vi "j_GetJoystickSignal.vi"(5 "RelJoyPos In":T1, 6 "NewJoystButtInfo":T2, 7 "NewJoystAxisInfo":T4, 8 "OldJoystButtInfo":T2, 9 "OldJoystickOffset":T3) -> (0 "MoveZ":bool, 1 "MoveXY":bool, 2 "Joystick Offset":T3, 3 "RelJoyPos":T1, 4 "TalkToMotors?":bool)   [LabVIEW 2014]
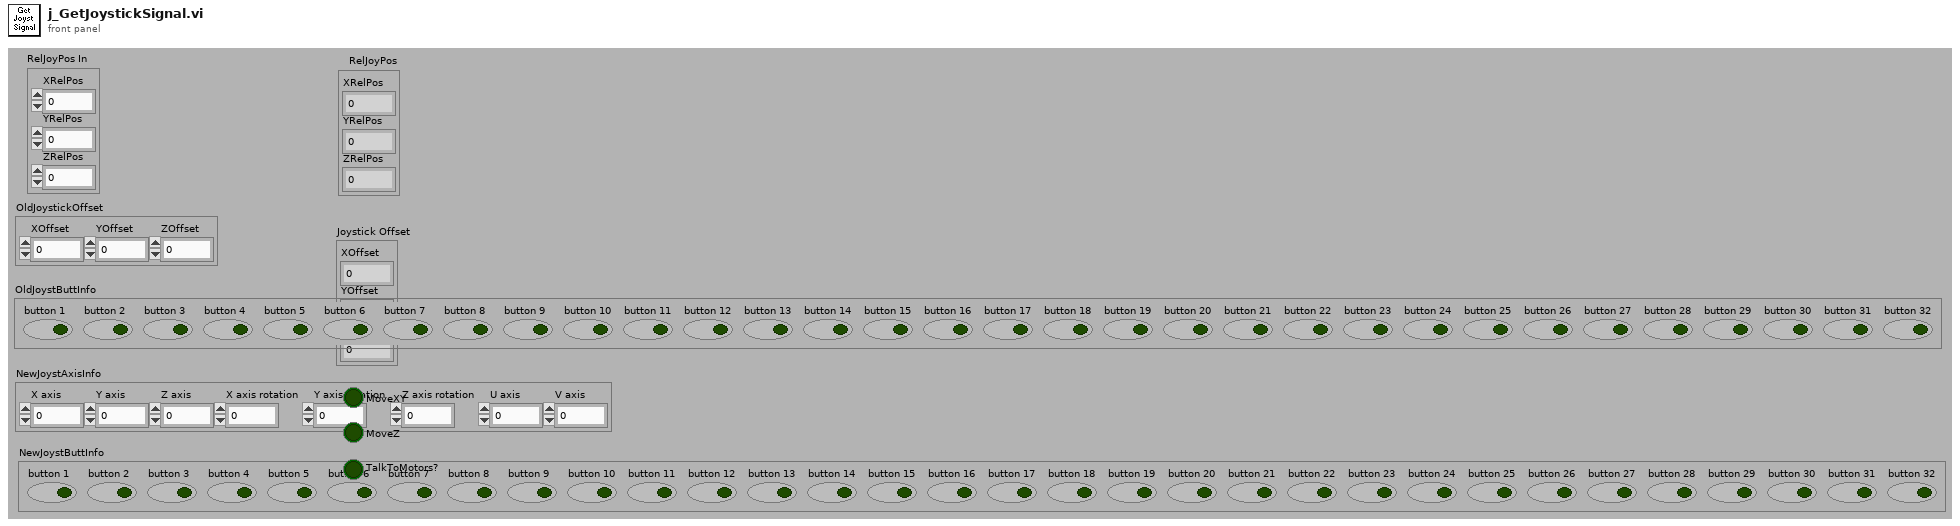
[diagram p1: front panel]
types:
  T1 = cluster{"XRelPos":i32, "YRelPos":i32, "ZRelPos":i32}
  T2 = cluster{"button 1":bool, "button 2":bool, "button 3":bool, "button 4":bool, "button 5":bool, "button 6":bool, "button 7":bool, "button 8":bool, "button 9":bool, "button 10":bool, "button 11":bool, "button 12":bool, "button 13":bool, "button 14":bool, "button 15":bool, "button 16":bool, "button 17":bool, "button 18":bool, "button 19":bool, "button 20":bool, "button 21":bool, "button 22":bool, "button 23":bool, "button 24":bool, "button 25":bool, "button 26":bool, "button 27":bool, "button 28":bool, "button 29":bool, "button 30":bool, "button 31":bool, "button 32":bool}
  T3 = cluster{"XOffset":i32, "YOffset":i32, "ZOffset":i32}
  T4 = cluster{"X axis":i32, "Y axis":i32, "Z axis":i32, "X axis rotation":i32, "Y axis rotation":i32, "Z axis rotation":i32, "U axis":i32, "V axis":i32}
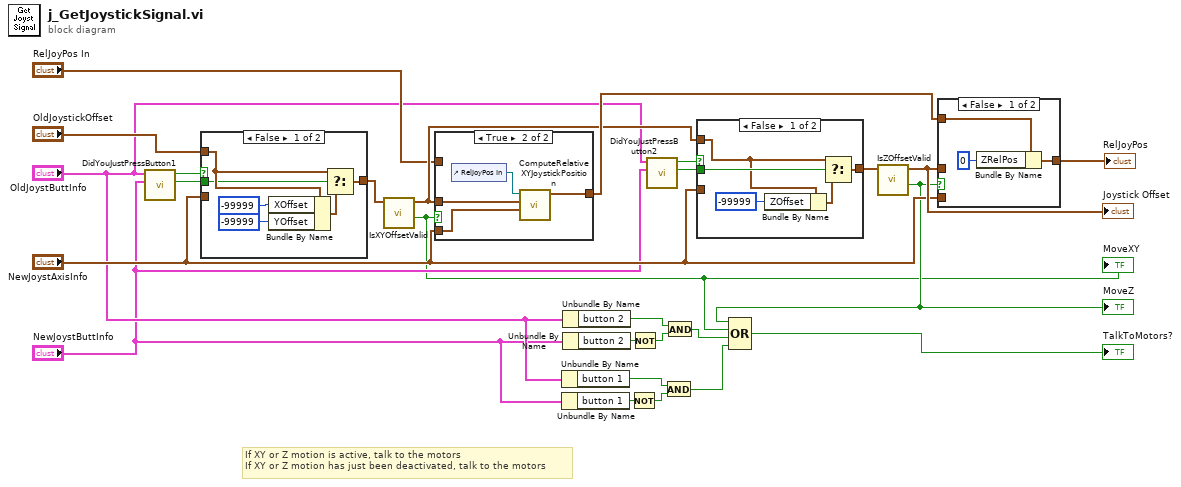
[diagram p0: block diagram]
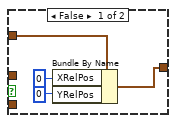
[diagram p2: hidden frame]
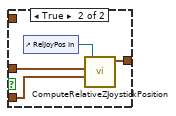
[diagram p3: hidden frame]
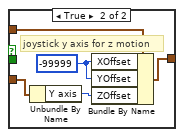
[diagram p4: hidden frame]
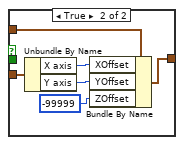
[diagram p5: hidden frame]
diagram:
  # "If XY or Z motion is active, talk to the motors\nIf XY or Z motion has just been deactivated, talk to the motors"
  n1 = call "DidYouJustPressButton1.vi"("New Button Info"="NewJoystButtInfo", "Old Button Info"="OldJoystButtInfo") -> ("Button1 New State"=w21:bool, "Did You Just Press Button1?"=w15:bool)  [unwired: 3 in, 1 out]
  n2 = case shown="False" w15 {
    tunnel: [w32 w38] -> w22
    tunnel: "NewJoystAxisInfo" -> [_ w35]
    tunnel: "OldJoystickOffset" -> [w31 w34]
    tunnel: w21 -> [w29 _]
    frame False {
      n3 = Bundle By Name(cluster=w31, "XOffset"=-99999, "YOffset"=-99999 ("XOffset")) -> (w30:T3)
      n4 = Select(t=w31, s=w29, f=w30) -> (s? t:f=w32:T3)
    }
    frame True {
      n5 = Unbundle By Name(w35) -> ("X axis"=w37:i32, "Y axis"=w36:i32)
      n6 = Bundle By Name(cluster=w34, "XOffset"=w37, "YOffset"=w36, "ZOffset"=-99999) -> (w38:T3)
    }
  }
  n7 = call "IsXYOffsetValid.vi"("Joystick Offset In"=w22) -> ("IsXYOffsetValid?"=w4:bool, "Joystick Offset"=w23:T3)  [unwired: 5 in]
  "MoveXY" <- w4
  n8 = case shown="True" w4 {
    tunnel: [w40 w44] -> w25
    tunnel: "NewJoystAxisInfo" -> [_ w46]
    tunnel: w23 -> [_ w45]
    tunnel: "RelJoyPos In" -> [w39 _]
    frame False {
      n9 = Bundle By Name(cluster=w39, "XRelPos"=0, "YRelPos"=0) -> (w40:T1)
    }
    frame True {
      n10 = control-ref of="RelJoyPos In"() -> (w43:refnum<vi>)
      n11 = call "ComputeRelativeXYJoystickPosition.vi"("Joystick Axis Info"=w46, "Joystick Offset"=w45, "reference"=w43) -> ("Rel XY Pos"=w44:T1)  [unwired: 4 in]
    }
  }
  n12 = Unbundle By Name("OldJoystButtInfo") -> ("button 1"=w9:bool)
  n13 = Unbundle By Name("NewJoystButtInfo") -> ("button 1"=w10:bool)
  n14 = Unbundle By Name("OldJoystButtInfo") -> ("button 2"=w12:bool)
  n15 = Unbundle By Name("NewJoystButtInfo") -> ("button 2"=w13:bool)
  n16 = Not(x=w10) -> (.not. x?=w8:bool)
  n17 = Not(x=w13) -> (.not. x?=w11:bool)
  n18 = call "DidYouJustPressButton2.vi"("New Button Info"="NewJoystButtInfo", "Old Button Info"="OldJoystButtInfo") -> ("Button2 New State"=w17:bool, "Did You Just Press Button2?"=w16:bool)  [unwired: 3 in, 1 out]
  n19 = And(x=w9, y=w8) -> (x .and. y?=w2:bool)
  n20 = And(x=w12, y=w11) -> (x .and. y?=w3:bool)
  n21 = case shown="False" w16 {
    tunnel: [w50 w56] -> w19
    tunnel: "NewJoystAxisInfo" -> [_ w55]
    tunnel: w17 -> [w51 _]
    tunnel: w23 -> [w49 w54]
    frame False {
      n22 = Bundle By Name(cluster=w49, "ZOffset"=-99999) -> (w47:T3)
      n23 = Select(t=w49, s=w51, f=w47) -> (s? t:f=w50:T3)
    }
    frame True {
      w52 = -99999 ("ZOffset")
      # "joystick y axis for z motion"
      n24 = Unbundle By Name(w55) -> ("Y axis"=w53:i32)
      n25 = Bundle By Name(cluster=w54, "XOffset"=w52, "YOffset"=w52, "ZOffset"=w53) -> (w56:T3)
    }
  }
  n26 = call "IsZOffsetValid.vi"("Joystick Offset In"=w19) -> ("IsZOffsetValid?"=w5:bool, "Joystick Offset"=w26:T3)  [unwired: 5 in]
  "Joystick Offset" <- w26
  "MoveZ" <- w5
  n27 = Compound Arithmetic op=OR(w5, w4, w3, w2) -> (→"TalkToMotors?":bool)
  n28 = case shown="False" w5 {
    tunnel: "NewJoystAxisInfo" -> [_ w63]
    tunnel: w26 -> [_ w62]
    tunnel: [w58 w61] -> w24
    tunnel: w25 -> [w57 _]
    frame False {
      n29 = Bundle By Name(cluster=w57, "ZRelPos"=0) -> (w58:T1)
    }
    frame True {
      n30 = control-ref of="RelJoyPos In"() -> (w60:refnum<vi>)
      n31 = call "ComputeRelativeZJoystickPosition.vi"("Joystick Axis Info"=w63, "Joystick Offset"=w62, "reference"=w60) -> ("Rel Z Pos"=w61:T1)  [unwired: 4 in]
    }
  }
  "RelJoyPos" <- w24
